vi "Read Server Stop.vi"(8 "error in (no error)":errorcluster, 11 "iService in":refnum<class "iService.lvclass">) -> (0 "error out":errorcluster, 2 "Server Stop":refnum<user-event>, 3 "iService out":refnum<class "iService.lvclass">)   [LabVIEW 2019, in "gRPC-servicer.lvlib" / "iService.lvclass"]
uses:
  iService.lvclass
  iService.lvclass/iService.ctl
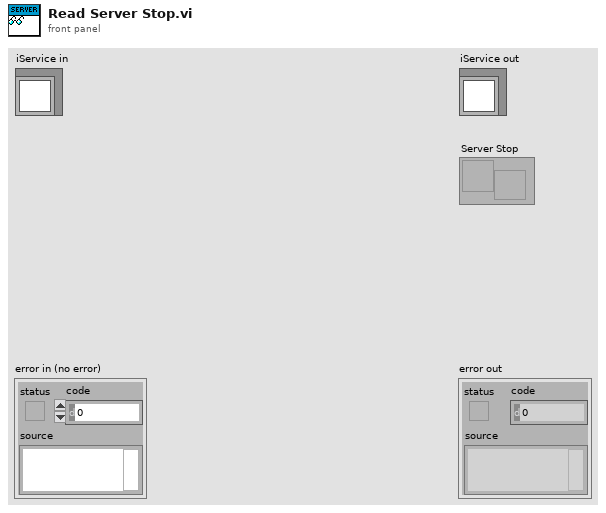
[diagram p1: front panel]
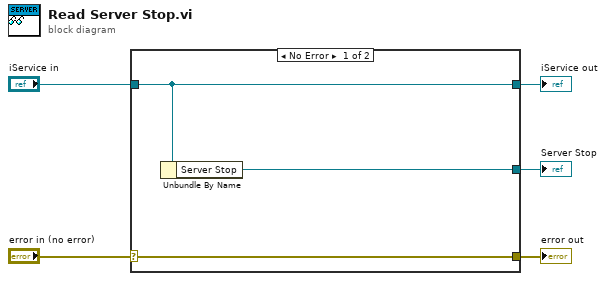
[diagram p0: block diagram]
diagram:
  n1 = case shown="No Error" "error in (no error)" {
    selector: "error in (no error)" -> [w8 w9]
    tunnel: [w8 w9] -> w4
    tunnel: [w7 w10] -> w2
    tunnel: "iService in" -> [w7 w10]
    tunnel: [w6 _] -> w1
    frame No Error {
      n2 = Unbundle By Name(w7) -> ("Server Stop"=w6:refnum<user-event>)
    }
    frame Error {
    }
  }
  "error out" <- w4
  "iService out" <- w2
  "Server Stop" <- w1
